vi "Update MemberTable In Panel.vi"(8 "error in (no error)":errorcluster, 10 "课程表":refnum<vi>, 11 "MemberTable in":refnum<class "TimeTable.lvclass">) -> (0 "error out":errorcluster, 3 "MemberTable out":refnum<class "TimeTable.lvclass">)   [LabVIEW 2015, in "Member_Actor.lvlib" / "TimeTable.lvclass"]
uses:
  TimeTable.lvclass
  TimeTable.lvclass/TimeTable.ctl
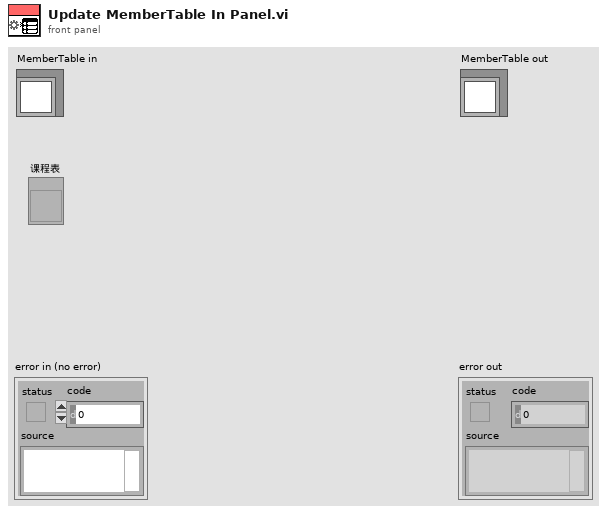
[diagram p1: front panel]
types:
  T1 = typedef "Member_Actor.lvlib/TimeTable.lvclass/Table_Cell.ctl" = cluster{"结束周":i32, "起始周":i32, "课程名称":string}
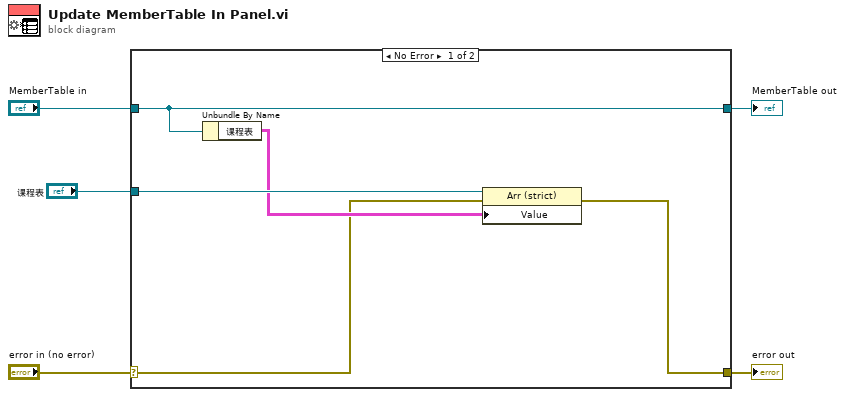
[diagram p0: block diagram]
diagram:
  n1 = case shown="No Error" "error in (no error)" {
    selector: "error in (no error)" -> [w7 w12]
    tunnel: [w6 w12] -> w4
    tunnel: [w9 w11] -> w2
    tunnel: "MemberTable in" -> [w9 w11]
    tunnel: "课程表" -> [w10 _]
    frame No Error {
      n2 = Unbundle By Name(w9) -> ("课程表"=w8:T1[][])
      n3 = property class="Arr (strict)"(reference=w10, error in=w7, "Value"=w8) -> (error out=w6:errorcluster)  [unwired: 1 out]
    }
    frame Error {
    }
  }
  "error out" <- w4
  "MemberTable out" <- w2
